vi "publish -- magnet field -- eventful.vi"(0 "freq  (Hz)":dbl=1000.0 format="%#_10f", 1 "publisher action":T2, 5 "gamma  (Hz)":dbl=1000.0, 7 "Voltage  (V)":cdb=1.133070214302279+0.0i) -> (4 "freq out (Hz)":dbl=1000.0 format="%#_10f", 6 "gamma OUT (Hz)":dbl=1000.0, 8 "Voltage out (V)":cdb=1.133070214302279+0.0i, 10 "response OUT":refnum<user-event>, 14 "response type":T1={"freq (Hz)"=1000.0, "gamma (Hz)"=1000.0, "Voltage (V)"=1.133070214302279+0.0i}, 15 "request event":refnum<user-event>)   [LabVIEW 2018]
uses:
  publisher action.ctl
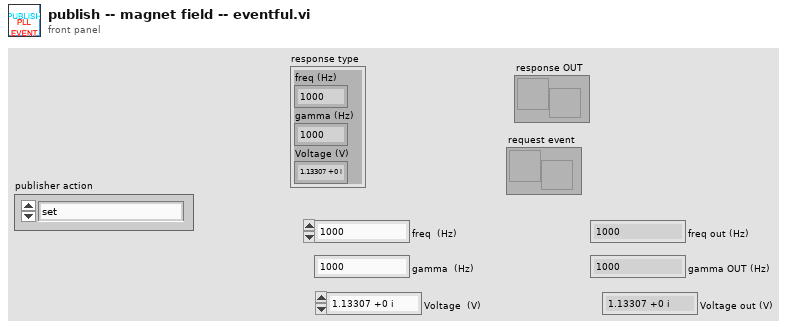
[diagram p1: front panel]
types:
  T1 = cluster{"freq (Hz)":dbl, "gamma (Hz)":dbl, "Voltage (V)":cdb}
  T2 = typedef "publisher action.ctl" = enum16{"set", "get", "init", "check"}
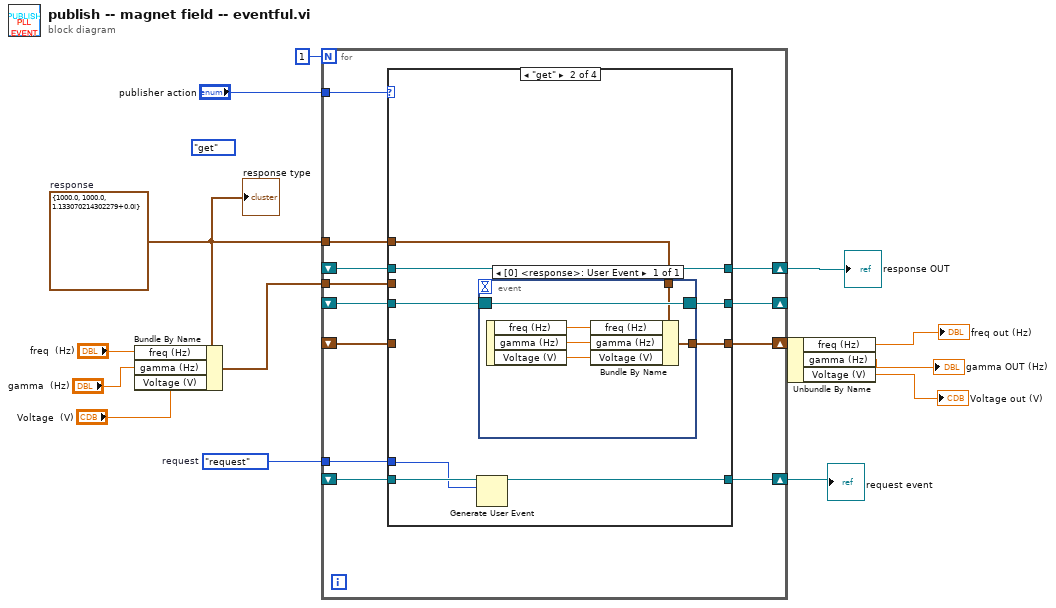
[diagram p0: block diagram]
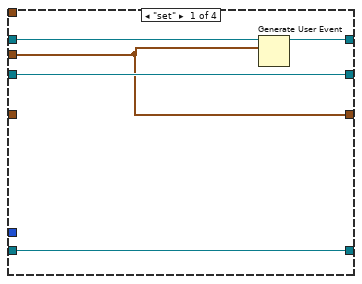
[diagram p2: hidden frame]
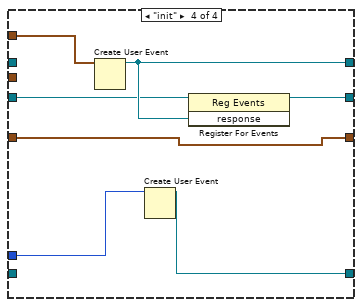
[diagram p4: hidden frame]
diagram:
  w9 = T1 {"freq (Hz)"=1000.0, "gamma (Hz)"=1000.0, "Voltage (V)"=1.133070214302279+0.0i}  # response
  w12 = enum16{"request"}."request"  # request
  (unwired) publisher_action."get" ("publisher action")
  n1 = Bundle By Name(cluster=w9, "freq (Hz)"="freq  (Hz)", "gamma (Hz)"="gamma  (Hz)", "Voltage (V)"="Voltage  (V)") -> (w5:T1)
  n2 = for {
    N: 1 -> [_]
    tunnel: "publisher action" -> [w26]
    tunnel: w5 -> [w25]
    shift-right: [w15] -> w4
    shift-left: _ -> [w24]
    shift-right: [w17] -> w10
    shift-left: _ -> [w16]
    shift-right: [w18] -> w11
    shift-left: _ -> [w23]
    shift-right: [w22] -> _
    shift-left: _ -> [w21]
    tunnel: w12 -> [w20]
    tunnel: w9 -> [w19]
    n3 = case shown="\"get\"" w26 {
      tunnel: w25 -> [w27 _ _ _]
      tunnel: w24 -> [_ _ w46 w50]
      tunnel: w16 -> [w29 w34 w47 _]
      tunnel: w23 -> [w30 w37 w48 _]
      tunnel: [w31 w39 w49 w52] -> w22
      tunnel: w21 -> [w31 w38 w49 w51]
      tunnel: w20 -> [_ w36 _ w55]
      tunnel: w19 -> [_ w33 _ w56]
      tunnel: [w30 w35 w48 w54] -> w18
      tunnel: [w28 w34 w47 w53] -> w17
      tunnel: [w27 w32 w46 w50] -> w15
      frame "set" {
        n4 = Generate User Event(user event=w29, event data cluster=w27) -> (user event out=w28:refnum<user-event>)  [unwired: 2 in, 1 out]
      }
      frame "get" {
        n5 = Generate User Event(user event=w37, event data cluster=w36) -> (user event out=w35:refnum<user-event>)  [unwired: 2 in, 1 out]
        n6 = event shown="[0] <response>: User Event" {
          selector: w38 -> [w45]
          dyn-events: [w45] -> w39
          timeout: _ -> [_]
          tunnel: w33 -> [w41]
          tunnel: [w40] -> w32
          event User Event {
            n7 = event-data() -> ("freq (Hz)"=w44:dbl, "gamma (Hz)"=w43:dbl, "Voltage (V)"=w42:cdb)  [unwired: 1 in]
            n8 = Bundle By Name(cluster=w41, "freq (Hz)"=w44, "gamma (Hz)"=w43, "Voltage (V)"=w42) -> (w40:T1)
          }
        }
      }
      frame "check", Default {
      }
      frame "init" {
        n9 = Create User Event(user event datatype=w56) -> (user event=w53:refnum<user-event>)  [unwired: 1 in, 1 out]
        n10 = Create User Event(user event datatype=w55) -> (user event=w54:refnum<user-event>)  [unwired: 1 in, 1 out]
        n11 = register-events(reference=w51, w53) -> (reference out=w52:refnum<event-registration>)  [unwired: 1 in, 1 out]
      }
    }
  }
  "request event" <- w11
  "response OUT" <- w10
  n12 = Unbundle By Name(w4) -> ("freq (Hz)"=→"freq out (Hz)":dbl, "gamma (Hz)"=→"gamma OUT (Hz)":dbl, "Voltage (V)"=→"Voltage out (V)":cdb)
  "response type" <- w9
